vi "Set_velocity.vi"(8 "error in (no error)":errorcluster, 10 "Set Velocity (mm/s)":dbl, 11 "Lifter_motor in":refnum<class "Lifter_motor.lvclass">) -> (0 "error out":errorcluster, 3 "Lifter_motor out":refnum<class "Lifter_motor.lvclass">)   [LabVIEW 2019, in "Lifter_motor.lvclass"]
uses:
  Lifter_motor.lvclass
  Lifter_motor.lvclass/Lifter_motor.ctl
  TCP Class/LifterTCP.lvclass
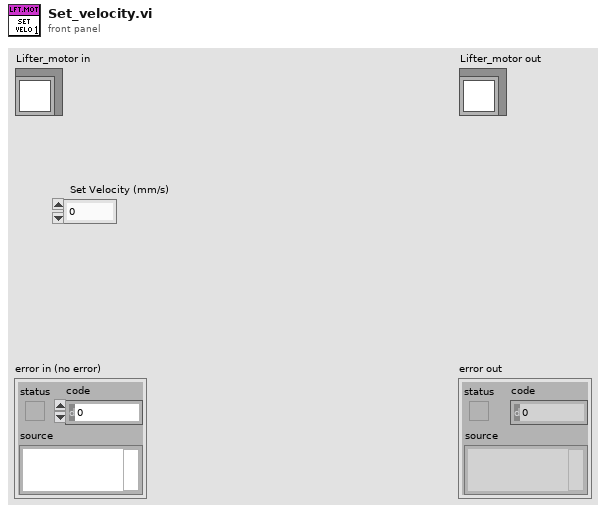
[diagram p1: front panel]
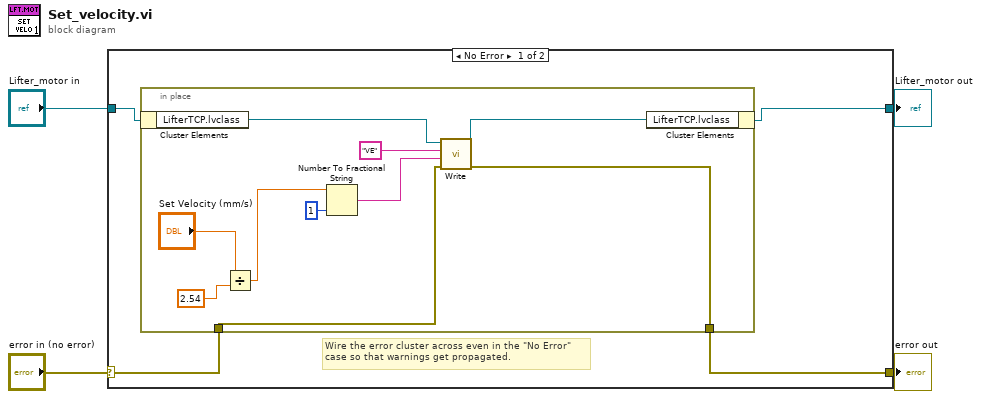
[diagram p0: block diagram]
diagram:
  n1 = case shown="No Error" "error in (no error)" {
    selector: "error in (no error)" -> [w8 w20]
    tunnel: [w7 w20] -> w3
    tunnel: [w6 w19] -> w1
    tunnel: "Lifter_motor in" -> [w5 w19]
    frame No Error {
      # "Wire the error cluster across even in the \"No Error\"\ncase so that warnings get propagated."
      n2 = in-place {
        in-place-border: [w15] -> w7
        in-place-border: w8 -> [w9]
        n3 = in-place-cluster #1(w5) -> ("LifterTCP.lvclass"=w18:refnum<class "LifterTCP.lvclass">)
        n4 = Divide(x="Set Velocity (mm/s)", y=2.54 ("x")) -> (x/y=w11:dbl)
        n5 = Number To Fractional String(number=w11, precision (6)=i16 1) -> (F-format string=w13:string)  [unwired: 2 in]
        n6 = call "Write.vi"("error in (no error)"=w9, "Parameter 2"=w13, "Parameter 1"="VE", "LifterTCP in"=w18) -> ("error out"=w15:errorcluster, "LifterTCP out"=w17:refnum<class "LifterTCP.lvclass">)  [unwired: 5 in, 1 out]
        n7 = in-place-cluster #1("LifterTCP.lvclass"=w17) -> (w6:refnum<class "Lifter_motor.lvclass">)
      }
    }
    frame Error {
    }
  }
  "error out" <- w3
  "Lifter_motor out" <- w1
